vi "Teleop.vi"(10 "Match Info":T2={"Autonomous Elapsed Seconds"=0.0, "TeleOp Elapsed Seconds"=0.0, "Disabled Elapsed Seconds"=0.0, "Visited Autonomous"=FALSE, "Visited TeleOp"=FALSE, "Visited Disabled"=FALSE, "Autonomous Settings"={"Autonomous Style"=enum."Independent", "VI Refnum"=refnum}}, 11 "Call Context":T3) -> ()   [LabVIEW 2019]
doc: "This VI is called for each TeleOp packet received from the DS where the robot is not disabled. It is often used to read from the joysticks and update I/O or to update setpoints for timed control loops. It should complete and return within 20 milliseconds or it may miss DS packets."
uses:
  <vilib>/Rock Robotics/WPI/DriverStation/WPI_DriverStationDerivedRobotMode.ctl
  <vilib>/Rock Robotics/WPI/DriverStation/WPI_DriverStationMatch Info.ctl
  <vilib>/addons/control/pid/autopid.llb/PID autotuning parameters (adv).ctl
  <vilib>/Rock Robotics/WPI/Utilities/WPI_GetSetVariantRefNum.vi
  <vilib>/Rock Robotics/Network Tables/NT Write Boolean Array.vi
  <vilib>/Rock Robotics/Network Tables/NT Write Numeric Array.vi
  <vilib>/Rock Robotics/Network Tables/NT Read Boolean.vi
  <vilib>/Rock Robotics/Network Tables/NT Read Number.vi
  <vilib>/addons/control/pid/NI_PID_autopid.lvlib
panel:
  out "tuning completed?":bool
  out "tuned PID gains":T1={"proportional gain (Kc)"=1.0, "integral time (Ti, min)"=0.01, "derivative time (Td, min)"=0.0} {"derivative time (Td, min)" format="%#.6g"; "integral time (Ti, min)" format="%#.6g"; "proportional gain (Kc)" format="%#.6g"}
  out "x/y":dbl
  in  "PID gains":T1={"proportional gain (Kc)"=0.038972, "integral time (Ti, min)"=0.119778, "derivative time (Td, min)"=0.028747} {"derivative time (Td, min)" format="%.6f"; "integral time (Ti, min)" format="%.6f"; "proportional gain (Kc)" format="%.6f"}
  in  "On":bool
  out "Yaw":dbl
  out "Sample Slider 0":dbl(slide) scale=0.0..5.0
  out "Sample Boolean 1":bool
  out "Sample Boolean 0":bool
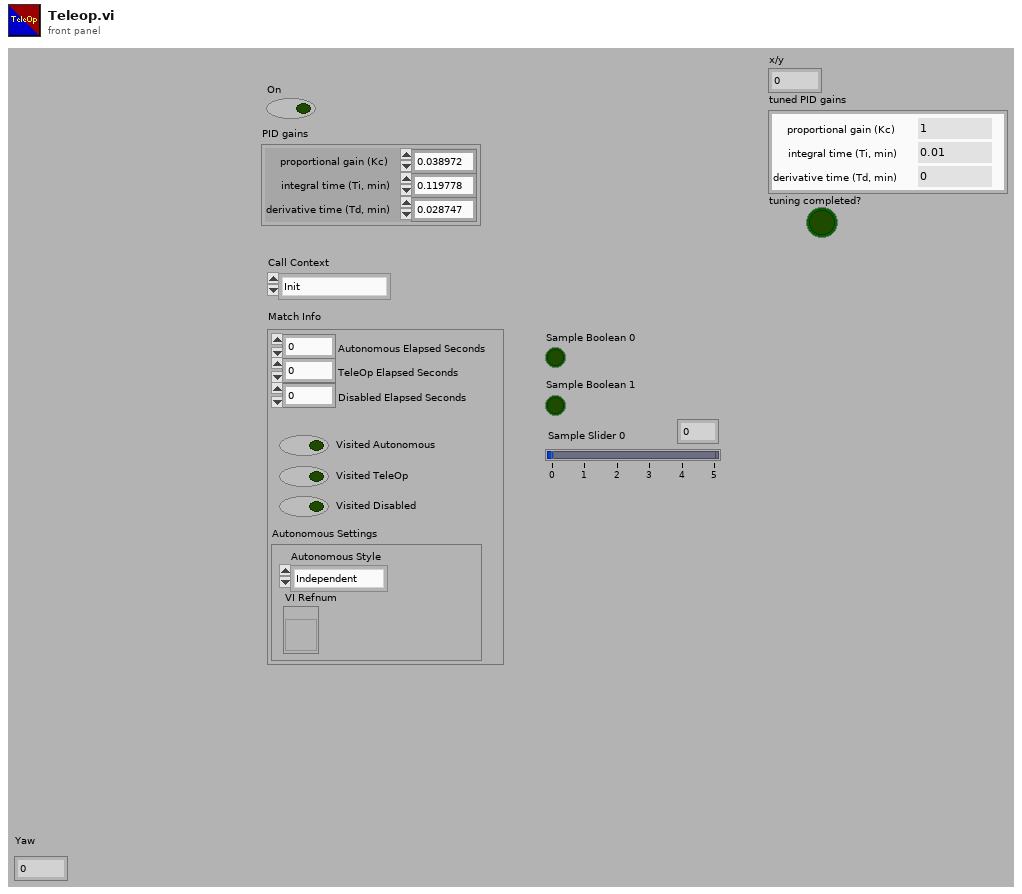
[diagram p1: front panel]
types:
  T1 = cluster{"proportional gain (Kc)":dbl, "integral time (Ti, min)":dbl, "derivative time (Td, min)":dbl}
  T2 = typedef "WPI_DriverStationMatch Info.ctl" = cluster{"Autonomous Elapsed Seconds":dbl, "TeleOp Elapsed Seconds":dbl, "Disabled Elapsed Seconds":dbl, "Visited Autonomous":bool, "Visited TeleOp":bool, "Visited Disabled":bool, "Autonomous Settings":cluster{"Autonomous Style":enum16{"Iterative", "Independent"}, "VI Refnum":refnum<vi>}}
  T3 = typedef "WPI_DriverStationDerivedRobotMode.ctl" = enum16{"Init", "Execute", "Stop"}
  T4 = typedef "NI_PID_autopid.lvlib/PID autotuning parameters (adv).ctl" = cluster{"technique":u16, "type of controller":u16, "control specification":u16, "amplitude":dbl}
  T5 = typedef "WPI_EncoderDevRef.ctl" = cluster{"DevStatus":errorcluster, "EncoderIndex":T6, "CounterIndex":T7, "DistancePerCount":dbl, "Decoding Type":T8}
  T6 = typedef "FPGA_EncoderIdx.ctl" = enum8{"Enc 0", "Enc 1", "Enc 2", "Enc 3", "Enc 4", "Enc 5", "Enc 6", "Enc 7", "Invalid"}
  T7 = typedef "FPGA_CounterCtrSystemIndex.ctl" = enum8{"Ctr 0", "Ctr 1", "Ctr 2", "Ctr 3", "Ctr 4", "Ctr 5", "Ctr 6", "Ctr 7", "Invalid"}
  T8 = typedef "WPI_EncoderType.ctl" = enum16{"1x", "2x", "4x"}
  T9 = typedef "WPI_MotorControlDeviceRef.ctl" = cluster{"DeviceStatus":errorcluster, "Type":T10, "PWM":cluster{"PWM Channel":T11, "DeadBand":T12}, "CAN":cluster{"Device Number":u8, "SetOutput VI Ref":variant, "GetOutput VI Ref":variant, "Enable VI Ref":variant, "Disable VI Ref":variant, "Data":variant}, "Invert":bool, "DIO PWM":cluster{"PWM \"Enable\" Channel":T11, "DIOChannel":T13, "PWM Rate":dbl}}
  T10 = typedef "WPI_MotorControlType.ctl" = enum16{"PWM", "CAN", "DIO PWM"}
  T11 = typedef "FPGA_DIOPWMChannel.ctl" = enum8{"PWM 0", "PWM 1", "PWM 2", "PWM 3", "PWM 4", "PWM 5", "PWM 6", "PWM 7", "PWM 8", "PWM 9", "PWM MXP 0", "PWM MXP 1", "PWM MXP 2", "PWM MXP 3", "PWM MXP 4", "PWM MXP 5", "PWM MXP 6", "PWM MXP 7", "PWM MXP 8", "PWM MXP 9", "Invalid"}
  T12 = typedef "WPI_PWMDeadband.ctl" = cluster{"Name":string, "maxPositivePwm":i32, "minPositivePwm":i32, "centerPwm":i32, "maxNegativePwm":i32, "minNegativePwm":i32, "angularRange":u16}
  T13 = typedef "FPGA_DIOChannel.ctl" = enum8{"DIO 0", "DIO 1", "DIO 2", "DIO 3", "DIO 4", "DIO 5", "DIO 6", "DIO 7", "DIO 8", "DIO 9", "DIO MXP 0", "DIO MXP 1", "DIO MXP 2", "DIO MXP 3", "DIO MXP 4", "DIO MXP 5", "DIO MXP 6", "DIO MXP 7", "DIO MXP 8", "DIO MXP 9", "DIO MXP 10", "DIO MXP 11", "DIO MXP 12", "DIO MXP 13", "DIO MXP 14", "DIO MXP 15", "SPI Port CS1", "SPI Port CS2", "SPI Port CS3", "SPI Port MISO", "SPI Port MOSI", "Invalid"}
  T14 = typedef "WPI_RobotDriveDevRef.ctl" = cluster{"DevStatus":errorcluster, "Motors[]":T9[], "Square Inputs":bool, "Max Output":dbl}
  T15 = typedef "WPI_JoystickDevRef.ctl" = cluster{"Device":T16}
  T16 = typedef "WPI_JoystickDeviceEnum.ctl" = enum16{"USB 0", "USB 1", "USB 2", "USB 3", "USB 4", "USB 5"}
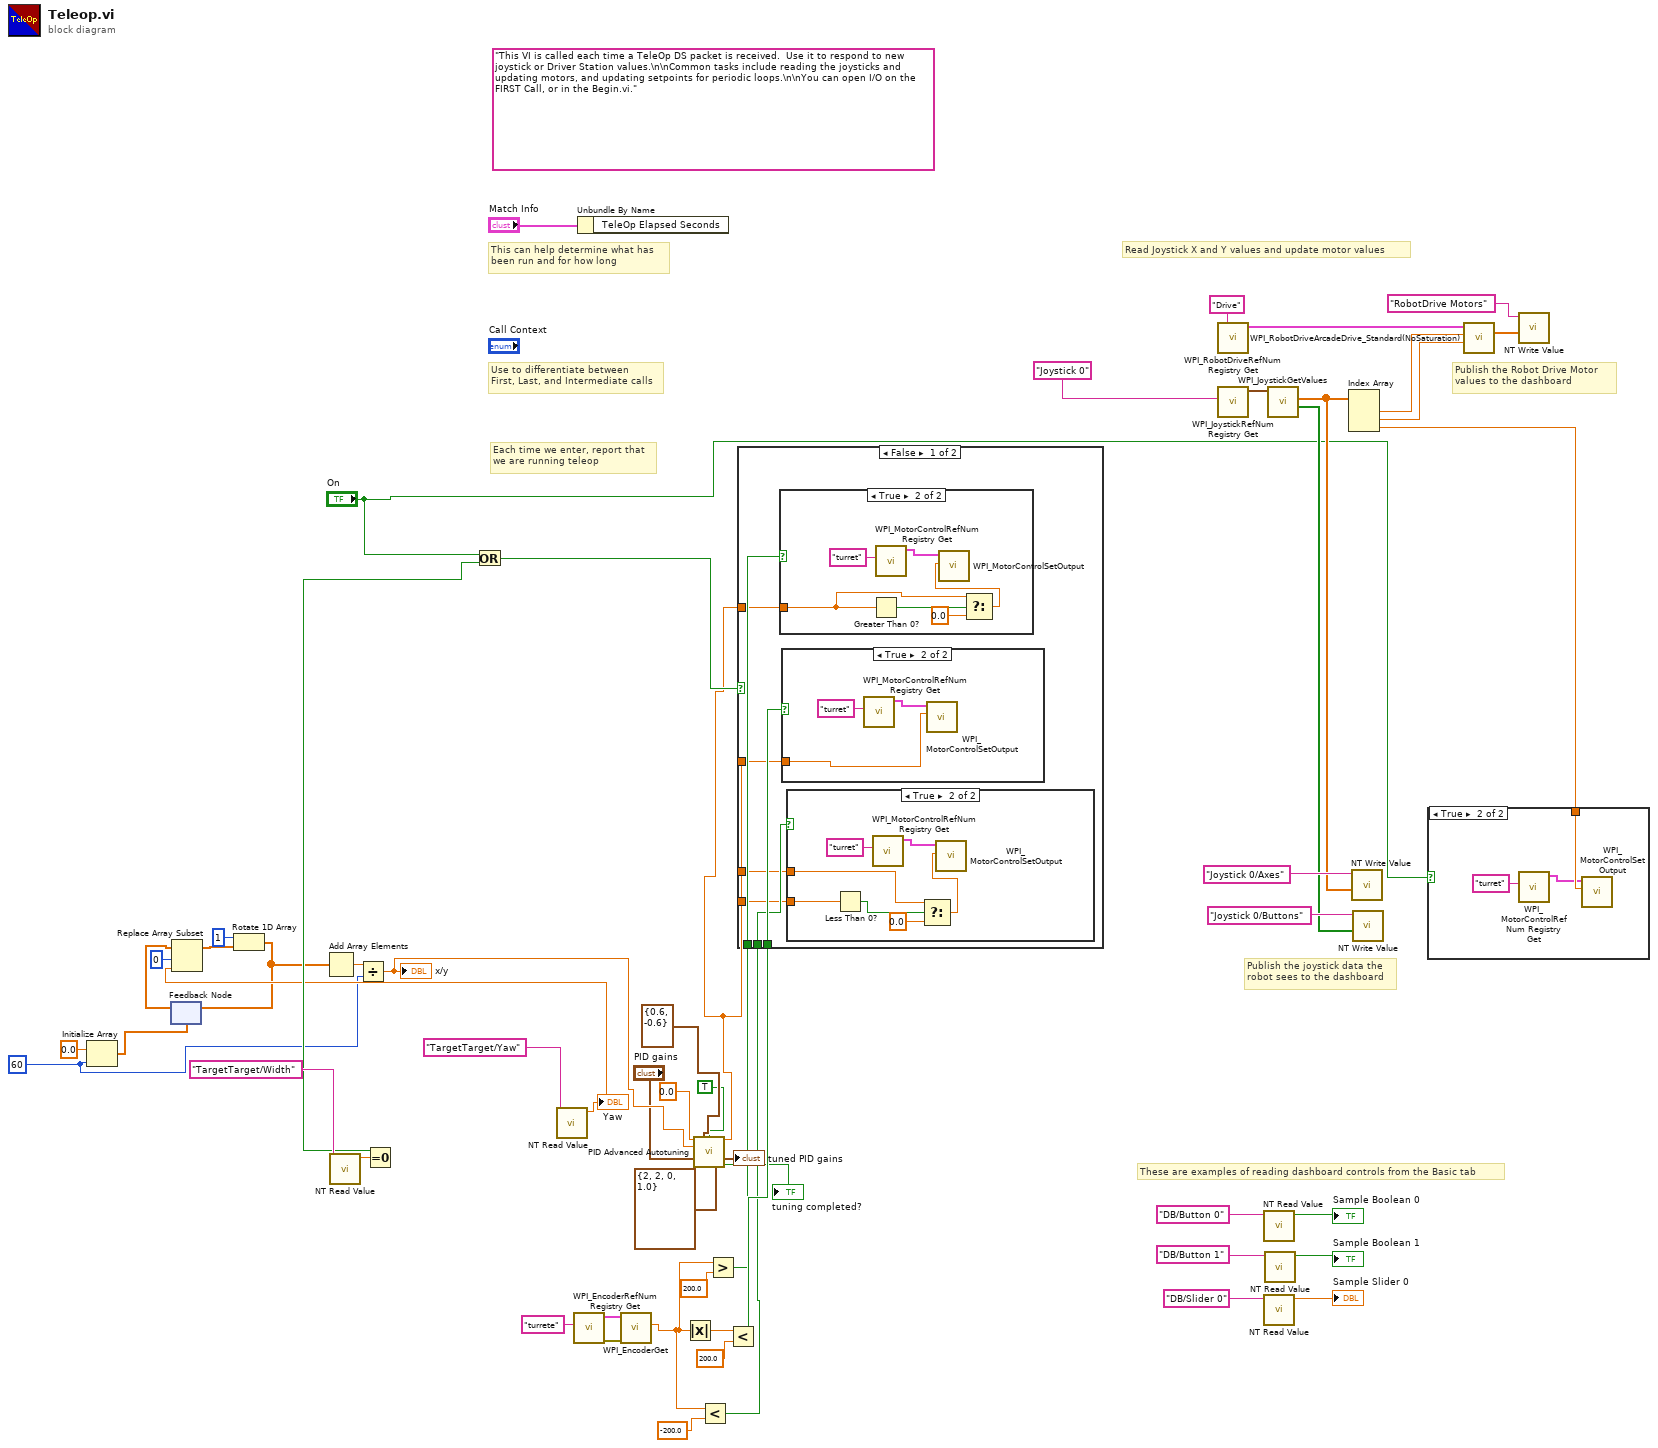
[diagram p0: block diagram]
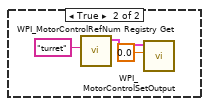
[diagram p5: hidden frame]
diagram:
  w10 = 60 ("dimension size")
  (unwired) "This VI is called each time a TeleOp DS packet is received.  Use it to respond to new joystick or Driver Station values.\n\nCommon tasks include reading the joysticks and updating motors, and updating setpoints for periodic loops.\n\nYou can open I/O on the FIRST Call, or in the Begin.vi."
  # "These are examples of reading dashboard controls from the Basic tab"
  # "Publish the Robot Drive Motor\nvalues to the dashboard"
  # "Publish the joystick data the\nrobot sees to the dashboard"
  # "Each time we enter, report that\nwe are running teleop"
  # "Use to differentiate between\nFirst, Last, and Intermediate calls"
  # "This can help determine what has\nbeen run and for how long"
  # "Read Joystick X and Y values and update motor values"
  n1 = Initialize Array(0.0 ("element"), w10) -> (w13:dbl[])
  n2 = feedback #1(w13) -> (w14:dbl[])
  n3 = call-poly <vilib>:"NT Read Value.vi"("Name"="TargetTarget/Width") -> ("Numeric"=w31:dbl)  [unwired: 9 in, 1 out]
  n4 = Equal To 0?(x=w31) -> (x = 0?=w30:bool)
  n5 = Or(x="On", y=w30) -> (x .or. y?=w20:bool)
  n6 = call-poly <vilib>:"NT Read Value.vi"("Name"="TargetTarget/Yaw") -> ("Numeric"=w18:dbl)  [unwired: 9 in, 1 out]
  "Yaw" <- w18
  n7 = Replace Array Subset(array=w14, new element=w18, index=0) -> (w16:dbl[])
  n8 = Rotate 1D Array(1:w16, 2:1 ("n")) -> (0:w12:dbl[])
  n9 = feedback-in #1(w12) -> ()
  n10 = Add Array Elements(numeric array=w12) -> (sum=w11:dbl)
  n11 = Divide(x=w11, y=w10) -> (x/y=w9:dbl)
  "x/y" <- w9
  n12 = call <vilib>:"WPI_EncoderRefNum Registry Get.vi"("refnum name"="turrete") -> ("error out"=w35:errorcluster, "EncoderDevRef"=w34:T5)  [unwired: 9 in]
  n13 = Unbundle By Name("Match Info") -> ()  [unwired: 1 out]
  n14 = call <vilib>:"WPI_EncoderGet.vi"("error in (no error)"=w35, "EncoderDevRef"=w34) -> ("Distance"=w21:dbl)  [unwired: 4 in, 5 out]
  n15 = Absolute Value(x=w21) -> (abs(x)=w28:dbl)
  n16 = call <vilib>:"PID Advanced Autotuning.vi"("setpoint"=0.0, "output range"=cluster{"output high":dbl, "output low":dbl} {"output high"=0.6, "output low"=-0.6}, "auto? (F)"=TRUE ("auto? (T)"), "process variable"=w9, "PID gains"="PID gains", "autotuning parameters"=T4 {"technique"=2, "type of controller"=2, "control specification"=0, "amplitude"=1.0}) -> ("output"=w6:dbl, "tuned PID gains"=→"tuned PID gains":T1, "tuning completed?"=→"tuning completed?":bool)  [unwired: 7 in]
  n17 = Less?(x=w21, y=-200.0) -> (x < y?=w24:bool)
  n18 = Greater?(x=w21, y=200.0) -> (0:w22:bool)
  n19 = Less?(x=w28, y=200.0) -> (x < y?=w26:bool)
  n20 = case shown="False" w20 {
    tunnel: w26 -> [w63 _]
    tunnel: w24 -> [w62 _]
    tunnel: w22 -> [w61 _]
    tunnel: w6 -> [w60 _]
    tunnel: w6 -> [w59 _]
    tunnel: w6 -> [w58 _]
    tunnel: w6 -> [w57 _]
    frame False {
      n21 = case shown="True" w61 {
        tunnel: w58 -> [_ w74]
        frame False {
        }
        frame True {
          n22 = Greater Than 0?(x=w74) -> (x > 0?=w78:bool)
          n23 = call <vilib>:"WPI_MotorControlRefNum Registry Get.vi"("refnum name"="turret") -> ("MotorControlDevRef"=w79:T9)  [unwired: 9 in, 1 out]
          n24 = Select(t=w74, s=w78, f=0.0) -> (s? t:f=w76:dbl)
          n25 = call <vilib>:"WPI_MotorControlSetOutput.vi"("Output"=w76, "MotorControlDevRef"=w79) -> ()  [unwired: 7 in, 3 out]
        }
      }
      n26 = case shown="True" w63 {
        tunnel: w60 -> [_ w71]
        frame False {
        }
        frame True {
          n27 = call <vilib>:"WPI_MotorControlRefNum Registry Get.vi"("refnum name"="turret") -> ("MotorControlDevRef"=w73:T9)  [unwired: 9 in, 1 out]
          n28 = call <vilib>:"WPI_MotorControlSetOutput.vi"("Output"=w71, "MotorControlDevRef"=w73) -> ()  [unwired: 7 in, 3 out]
        }
      }
      n29 = case shown="True" w62 {
        tunnel: w59 -> [_ w65]
        tunnel: w57 -> [_ w64]
        frame False {
        }
        frame True {
          n30 = Less Than 0?(x=w64) -> (x < 0?=w68:bool)
          n31 = call <vilib>:"WPI_MotorControlRefNum Registry Get.vi"("refnum name"="turret") -> ("MotorControlDevRef"=w70:T9)  [unwired: 9 in, 1 out]
          n32 = Select(t=w65, s=w68, f=0.0) -> (s? t:f=w66:dbl)
          n33 = call <vilib>:"WPI_MotorControlSetOutput.vi"("Output"=w66, "MotorControlDevRef"=w70) -> ()  [unwired: 7 in, 3 out]
        }
      }
    }
    frame True {
      n34 = call <vilib>:"WPI_MotorControlRefNum Registry Get.vi"("refnum name"="turret") -> ("MotorControlDevRef"=w82:T9)  [unwired: 9 in, 1 out]
      n35 = call <vilib>:"WPI_MotorControlSetOutput.vi"("Output"=0.0, "MotorControlDevRef"=w82) -> ()  [unwired: 7 in, 3 out]
    }
  }
  n36 = call <vilib>:"WPI_RobotDriveRefNum Registry Get.vi"("refnum name"="Drive") -> ("RobotDriveDevRef"=w54:T14)  [unwired: 1 in, 9 out]
  n37 = call <vilib>:"WPI_JoystickRefNum Registry Get.vi"("refnum name"="Joystick 0") -> ("JoystickDevRef"=w51:T15)  [unwired: 1 in, 9 out]
  n38 = call-poly <vilib>:"NT Read Value.vi"("Name"="DB/Button 0" ("refnum name")) -> ("Boolean"=→"Sample Boolean 0":bool)  [unwired: 9 in, 1 out]
  n39 = call-poly <vilib>:"NT Read Value.vi"("Name"="DB/Slider 0" ("refnum name")) -> ("Numeric"=→"Sample Slider 0":dbl)  [unwired: 9 in, 1 out]
  n40 = call-poly <vilib>:"NT Read Value.vi"("Name"="DB/Button 1" ("refnum name")) -> ("Boolean"=→"Sample Boolean 1":bool)  [unwired: 9 in, 1 out]
  n41 = call <vilib>:"WPI_JoystickGetValues.vi"("JoystickDevRef"=w51) -> ("Buttons"=w46:bool[], "Axes"=w47:dbl[])  [unwired: 6 in, 3 out]
  n42 = Index Array(array=w47) -> (element #1=w53:dbl, element #2=w50:dbl, element #3=w37:dbl)  [unwired: 3 in]
  n43 = call-poly <vilib>:"NT Write Value.vi"("Numeric Array"=w47, "Name"="Joystick 0/Axes") -> ()  [unwired: 9 in, 1 out]
  n44 = call-poly <vilib>:"NT Write Value.vi"("Boolean Array"=w46, "Name"="Joystick 0/Buttons") -> ()  [unwired: 9 in, 1 out]
  n45 = case shown="True" "On" {
    tunnel: w37 -> [_ w85]
    frame False {
    }
    frame True {
      n46 = call <vilib>:"WPI_MotorControlRefNum Registry Get.vi"("refnum name"="turret") -> ("MotorControlDevRef"=w84:T9)  [unwired: 9 in, 1 out]
      n47 = call <vilib>:"WPI_MotorControlSetOutput.vi"("Output"=w85, "MotorControlDevRef"=w84) -> ()  [unwired: 7 in, 3 out]
    }
  }
  n48 = call <vilib>:"WPI_RobotDriveArcadeDrive_Standard(NoSaturation).vi"("Y axis value"=w50, "X axis value"=w53, "RobotDriveDevRef"=w54) -> ("Motor Values"=w39:dbl[])  [unwired: 1 in, 7 out]
  n49 = call-poly <vilib>:"NT Write Value.vi"("Numeric Array"=w39, "Name"="RobotDrive Motors") -> ()  [unwired: 9 in, 1 out]
